vi "ELL9 Device Engine.vi"() -> ()   [LabVIEW 2020]
uses:
  FW Type Defs/FW Actions.ctl
  FW Type Defs/FW Notifier Type.ctl
  <vilib>/Instr/_visa.llb/VISA Configure Serial Port (Instr).vi
panel:
  out "FW ID":string
  in  "COM Port":string[](array[string])
  in  "Notifier Name":string="Not a Name"
  out "Current Position":u8
  in  "Quit":bool
  in  "Get Position":bool
  in  "FW Position":u8=1 min=1 max=8
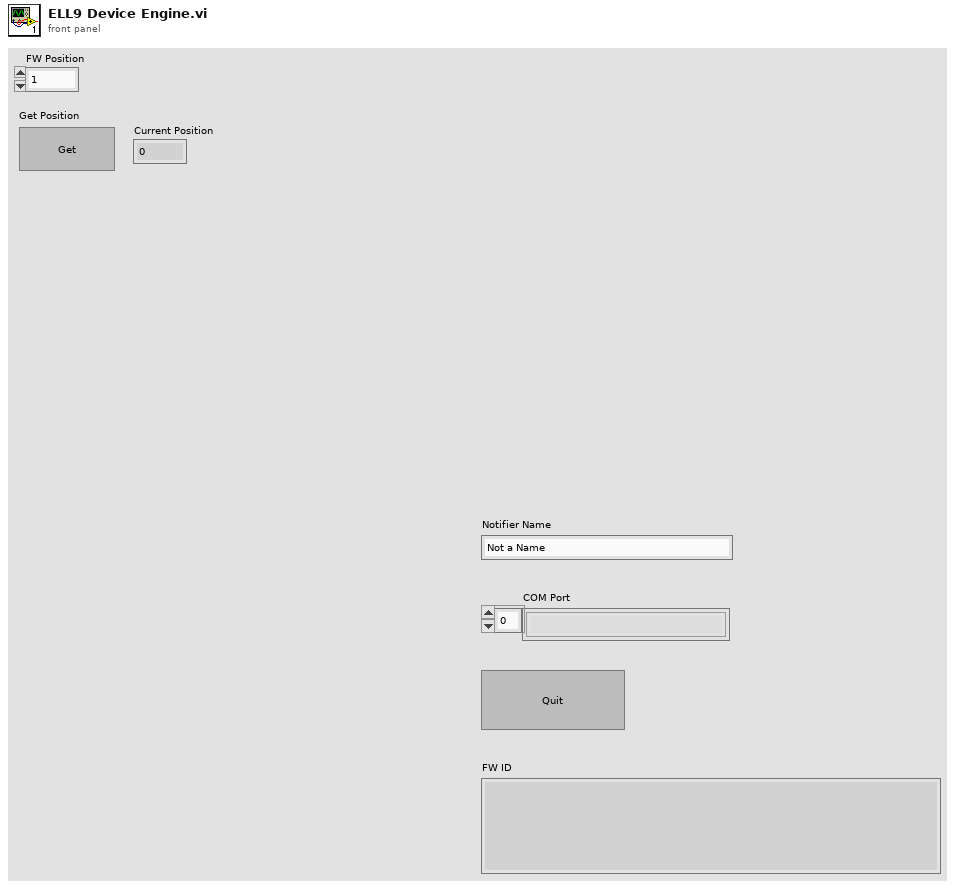
[diagram p1: front panel]
types:
  T1 = typedef "FW Notifier Type.ctl" = cluster{"Actions":T2, "Set Position":u8, "Actual Position":u8, "Speed":dbl, "Num Positions":u8, "Received":bool}
  T2 = typedef "FW Actions.ctl" = enum16{"Set Position", "Get Position", "Get Num Positions", "Set Speed", "Confirm Pos", "Quit"}
  T3 = enum32{"Invalid", "Standard", "Closed", "Hidden", "Minimized", "Maximized"}
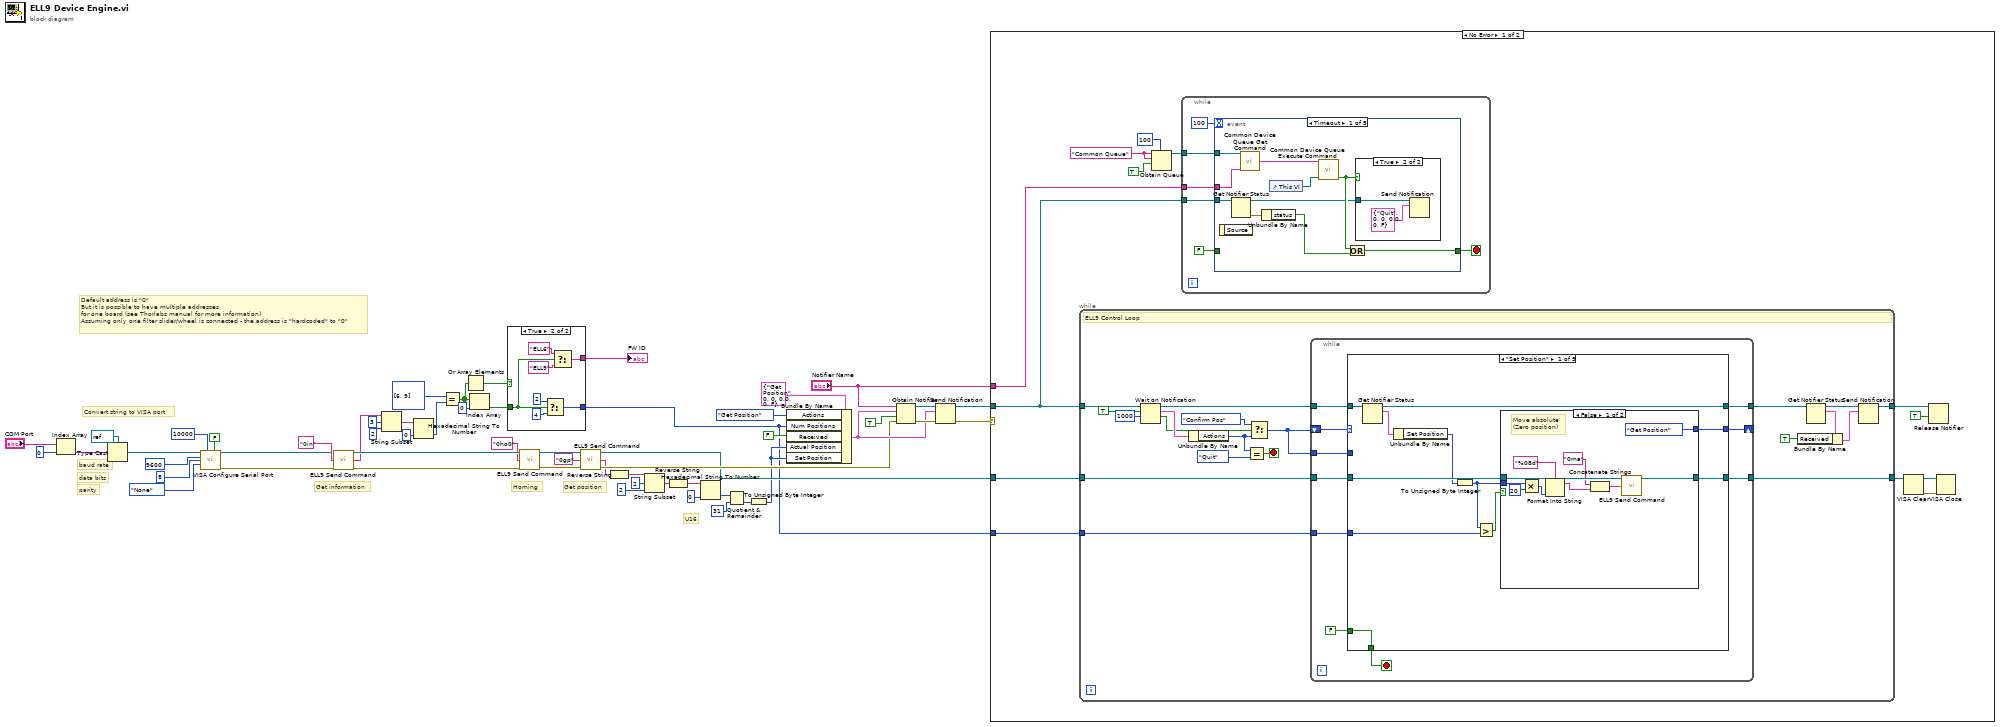
[diagram p0: block diagram]
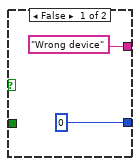
[diagram p2: hidden frame]
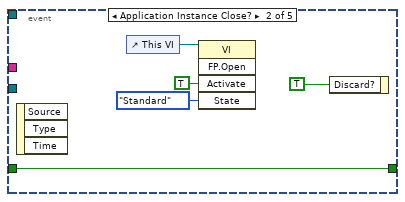
[diagram p4: hidden frame]
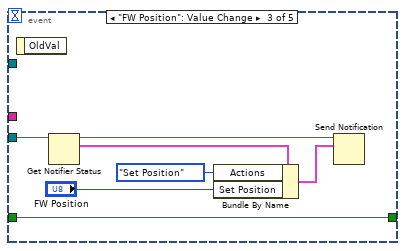
[diagram p5: hidden frame]
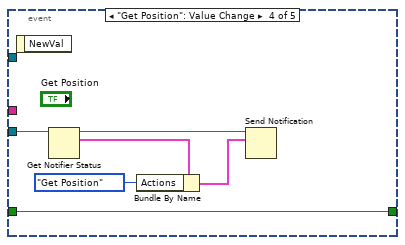
[diagram p6: hidden frame]
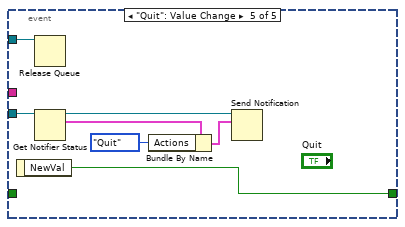
[diagram p7: hidden frame]
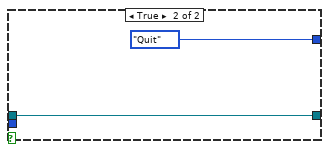
[diagram p8: hidden frame]
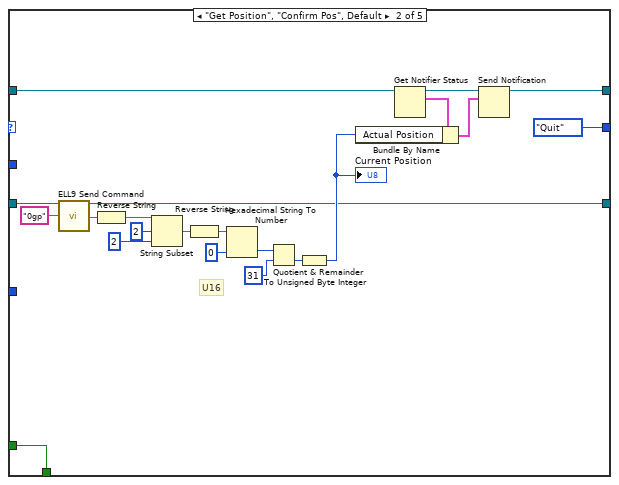
[diagram p9: hidden frame]
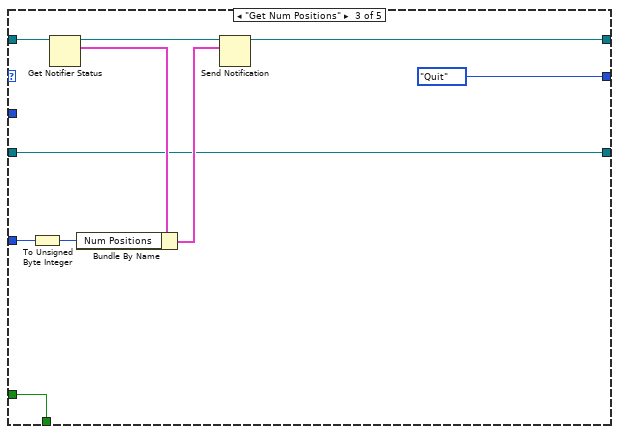
[diagram p10: hidden frame]
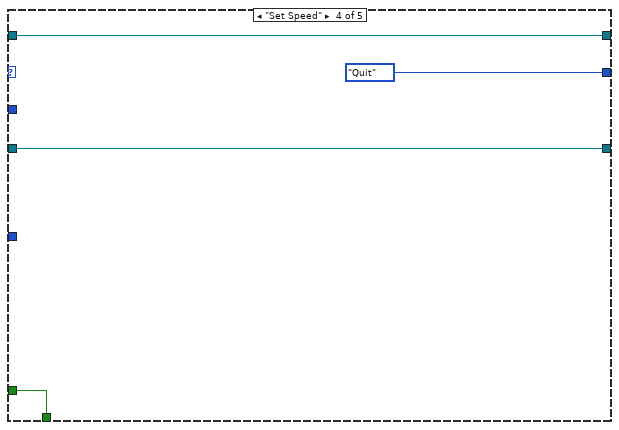
[diagram p11: hidden frame]
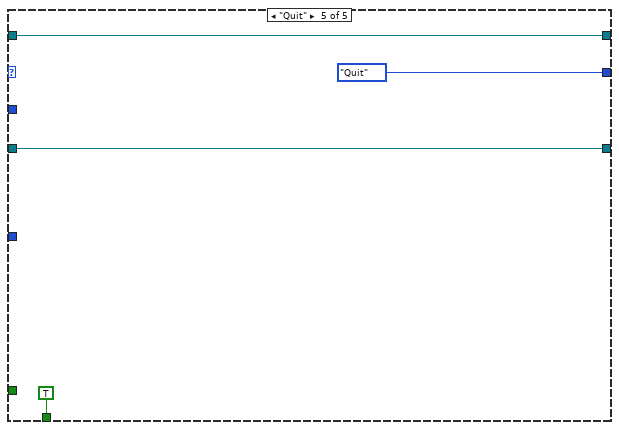
[diagram p12: hidden frame]
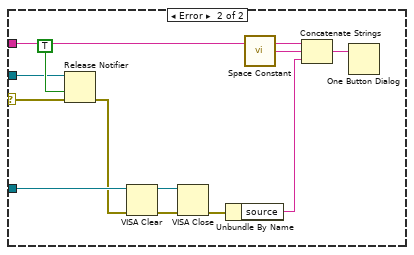
[diagram p13: hidden frame]
diagram:
  # "U16"
  # "Get position"
  # "Default address is \"0\"\nBut it is possible to have multiple addresses \nfor one board (see Thorlabs manual for more information)\nAssuming only one filter slider/wheel is connected - the address is \"hardcoded\" to \"0\""
  # "Get information"
  # "Homing"
  # "Convert string to VISA port"
  # "parity"
  # "data bits"
  # "baud rate"
  n1 = Index Array(array="COM Port", index=0) -> (element=w38:string)
  n2 = Type Cast(type=refnum<visa-resource-name> refnum ("VISA resource name"), x=w38) -> (*(type *) &x=w36:refnum<visa-resource-name>)
  n3 = call-poly "VISA Configure Serial Port"("VISA resource name"=w36, "timeout (10sec)"=u32 10000, "Enable Termination\nChar (T)"=FALSE ("Enable Termination\nChar (T)"), "baud rate (9600)"=u32 9600 ("nbaud"), "data bits (8)"=u16 8, "parity (0:none)"=enum16{"None", "Odd", "Even", "Mark", "Space"}."None") -> ("VISA resource name out"=w27:refnum<visa-resource-name>, "error out"=w1:errorcluster)  [unwired: 4 in, 4 out]
  n4 = call "ELL9 Send Command.vi"("VISA Ref"=w27, "Command"="0in" ("write buffer"), "Error In"=w1) -> ("VISA Ref Dup"=w33:refnum<visa-resource-name>, "Reply"=w5:string, "Error Out"=w34:errorcluster)  [unwired: 9 in, 1 out]
  n5 = String Subset(string=w5, offset (0)=3, length (rest)=2 ("length (rest)")) -> (substring=w11:string)
  n6 = Hexadecimal String To Number(string=w11, default (0uL)=u16 0 ("default (0 U32)")) -> (number=w4:u16)  [unwired: 1 in, 1 out]
  n7 = Equal?(x=u16[] [6, 9] ("default (0 U32)"), y=w4) -> (x = y?=w9:bool[])
  n8 = Or Array Elements(Boolean array=w9) -> (logical OR=w10:bool)
  n9 = Index Array(array=w9, index=0) -> (element=w7:bool)
  n10 = case shown="True" w10 {
    tunnel: w7 -> [_ w61]
    tunnel: ["Wrong device" ("write buffer") w62] -> w6
    tunnel: [u8 0 ("default (0 U32)") w58] -> w2
    frame False {
    }
    frame True {
      n11 = Select(t=u8 2 ("default (0 U32)"), s=w61, f=u8 4 ("default (0 U32)")) -> (s? t:f=w58:u8)
      n12 = Select(t="ELL6" ("write buffer"), s=w61, f="ELL9" ("write buffer")) -> (s? t:f=w62:string)
    }
  }
  "FW ID" <- w6
  n13 = call "ELL9 Send Command.vi"("VISA Ref"=w33, "Command"="0ho0" ("write buffer"), "Error In"=w34) -> ("VISA Ref Dup"=w30:refnum<visa-resource-name>, "Error Out"=w31:errorcluster)  [unwired: 9 in, 2 out]
  n14 = call "ELL9 Send Command.vi"("VISA Ref"=w30, "Command"="0gp" ("write buffer"), "Error In"=w31) -> ("VISA Ref Dup"=w21:refnum<visa-resource-name>, "Reply"=w24:string, "Error Out"=w28:errorcluster)  [unwired: 9 in, 1 out]
  n15 = Reverse String(1:w24) -> (0:w23:string)
  n16 = String Subset(string=w23, offset (0)=2, length (rest)=2 ("length (rest)")) -> (substring=w22:string)
  n17 = Reverse String(1:w22) -> (0:w18:string)
  n18 = Hexadecimal String To Number(string=w18, default (0uL)=u16 0 ("default (0 U32)")) -> (number=w20:u16)  [unwired: 1 in, 1 out]
  n19 = Quotient & Remainder(x=w20, y=u16 31) -> (floor(x/y)=w16:u16)  [unwired: 1 out]
  n20 = To Unsigned Byte Integer(number=w16) -> (unsigned 8bit integer=w15:u8)
  n21 = Bundle By Name(cluster=T1 {"Actions"=enum."Get Position", "Set Position"=0, "Actual Position"=0, "Speed"=0.0, "Num Positions"=0, "Received"=FALSE} ("Note Type"), "Actions"=FW_Actions."Get Position", "Num Positions"=w2, "Received"=FALSE ("Received?"), "Actual Position"=w15, "Set Position"=w15) -> (w49:T1)
  n22 = Obtain Notifier(name (unnamed)="Notifier Name", notification data type=w49, create if not found? (T)=TRUE, error in (no error)=w28) -> (notifier out=w54:refnum<notifier>, error out=w53:errorcluster)  [unwired: 1 out]
  n23 = Send Notification(notification=w49, notifier=w54, error in (no error)=w53) -> (notifier out=w47:refnum<notifier>, error out=w48:errorcluster)
  n24 = case shown="No Error" w48 {
    selector: w48 -> [_ w222]
    tunnel: w47 -> [w75 w223]
    tunnel: "Notifier Name" -> [w74 w221]
    tunnel: w21 -> [w69 w214]
    tunnel: w2 -> [w68 _]
    frame No Error {
      w73 = "Common Queue" ("Unique Notifier Name")
      n25 = while {
        tunnel: w75 -> [w134]
        tunnel: [w135] -> w76
        tunnel: w69 -> [w130]
        tunnel: [w129] -> w65
        tunnel: w68 -> [w128]
        stop <- w140 stop-if-true
        # "ELL9 Control Loop"
        n26 = Wait on Notification(notifier=w134, ignore previous (F)=TRUE, timeout in ms (-1)=1000) -> (notifier out=w132:refnum<notifier>, notification=w127:T1, timed out?=w123:bool)  [unwired: 1 in, 1 out]
        n27 = Unbundle By Name(w127) -> ("Actions"=w124:T2)
        n28 = Equal?(x=w124, y=FW_Actions."Quit") -> (x = y?=w140:bool)
        n29 = Select(t=FW_Actions."Confirm Pos", s=w123, f=w124) -> (s? t:f=w122:T2)
        n30 = while {
          tunnel: w132 -> [w149]
          tunnel: [w148] -> w131
          tunnel: w130 -> [w145]
          tunnel: [w144] -> w129
          tunnel: w128 -> [w143]
          shift-right: [w142] -> _
          shift-left: w122 -> [w150]
          tunnel: w122 -> [w141]
          stop <- w146 stop-if-true
          n31 = case shown="\"Set Position\"" w150 {
            tunnel: w149 -> [w157 w193 w203 w208 w212]
            tunnel: [w156 w191 w201 w208 w212] -> w148
            tunnel: [w161 w194 w204 w206 TRUE] -> w146
            tunnel: FALSE -> [w161 w194 w204 w206 _]
            tunnel: w145 -> [w159 w187 w195 w205 w210]
            tunnel: [w155 w174 w195 w205 w210] -> w144
            tunnel: w143 -> [w152 _ w198 _ _]
            tunnel: [w160 FW_Actions."Quit" ("f") FW_Actions."Quit" ("f") FW_Actions."Quit" ("f") FW_Actions."Quit" ("f")] -> w142
            tunnel: w141 -> [_ _ _ _ _]
            frame "Set Position" {
              n32 = Get Notifier Status(notifier=w157) -> (notifier out=w156:refnum<notifier>, current notification=w158:T1)  [unwired: 1 in, 3 out]
              n33 = Unbundle By Name(w158) -> ("Set Position"=w154:u8)
              n34 = To Unsigned Byte Integer(number=w154) -> (unsigned 8bit integer=w153:u8)
              n35 = Greater?(x=w153, y=w152) -> (0:w151:bool)
              n36 = case shown="False" w151 {
                tunnel: [FW_Actions."Get Position" ("f") FW_Actions."Quit" ("f")] -> w160
                tunnel: w159 -> [w170 w173]
                tunnel: [w169 w173] -> w155
                tunnel: w153 -> [w168 _]
                frame False {
                  # "Move absolute\n(Zero position)"
                  n37 = Multiply(x=w168, y=u8 20) -> (x*y=w165:u8)
                  n38 = Format Into String(format string="%08d", w165) -> (resulting string=w164:string)  [unwired: 2 in, 1 out]
                  n39 = Concatenate Strings("0ma", w164) -> (w162:string)
                  n40 = call "ELL9 Send Command.vi"("VISA Ref"=w170, "Command"=w162) -> ("VISA Ref Dup"=w169:refnum<visa-resource-name>)  [unwired: 10 in, 3 out]
                }
                frame True {
                }
              }
            }
            frame "Get Position", "Confirm Pos", Default {
              # "U16"
              n41 = call "ELL9 Send Command.vi"("VISA Ref"=w187, "Command"="0gp" ("write buffer")) -> ("VISA Ref Dup"=w174:refnum<visa-resource-name>, "Reply"=w176:string)  [unwired: 10 in, 2 out]
              n42 = Reverse String(1:w176) -> (0:w183:string)
              n43 = String Subset(string=w183, offset (0)=2, length (rest)=2 ("length (rest)")) -> (substring=w182:string)
              n44 = Reverse String(1:w182) -> (0:w179:string)
              n45 = Hexadecimal String To Number(string=w179, default (0uL)=u16 0 ("default (0 U32)")) -> (number=w181:u16)  [unwired: 1 in, 1 out]
              n46 = Quotient & Remainder(x=w181, y=u16 31) -> (floor(x/y)=w177:u16)  [unwired: 1 out]
              n47 = To Unsigned Byte Integer(number=w177) -> (unsigned 8bit integer=w175:u8)
              "Current Position" <- w175
              n48 = Get Notifier Status(notifier=w193) -> (notifier out=w192:refnum<notifier>, current notification=w190:T1)  [unwired: 1 in, 3 out]
              n49 = Bundle By Name(cluster=w190, "Actual Position"=w175) -> (w189:T1)
              n50 = Send Notification(notification=w189, notifier=w192) -> (notifier out=w191:refnum<notifier>)  [unwired: 1 in, 1 out]
            }
            frame "Get Num Positions" {
              n51 = To Unsigned Byte Integer(number=w198) -> (unsigned 8bit integer=w197:u8)
              n52 = Get Notifier Status(notifier=w203) -> (notifier out=w202:refnum<notifier>, current notification=w199:T1)  [unwired: 1 in, 3 out]
              n53 = Bundle By Name(cluster=w199, "Num Positions"=w197) -> (w196:T1)
              n54 = Send Notification(notification=w196, notifier=w202) -> (notifier out=w201:refnum<notifier>)  [unwired: 1 in, 1 out]
            }
            frame "Set Speed" {
            }
            frame "Quit" {
            }
          }
        }
        n55 = Get Notifier Status(notifier=w131) -> (notifier out=w136:refnum<notifier>, current notification=w138:T1)  [unwired: 1 in, 3 out]
        n56 = Bundle By Name(cluster=w138, "Received"=TRUE ("Received?")) -> (w139:T1)
        n57 = Send Notification(notification=w139, notifier=w136) -> (notifier out=w135:refnum<notifier>)  [unwired: 1 in, 1 out]
      }
      n58 = Obtain Queue(max queue size (-1, unlimited)=100, name (unnamed)=w73, element data type=w73, create if not found? (T)=TRUE) -> (queue out=w70:refnum<queue>)  [unwired: 1 in, 2 out]
      n59 = while {
        tunnel: w70 -> [w83]
        tunnel: w75 -> [w80]
        tunnel: w74 -> [w78]
        stop <- w79 stop-if-true
        n60 = event shown="[0] Timeout" {
          selector: _ -> [_ _ _ _ _]
          dyn-events: _ -> [_ _ _ _ _]
          timeout: 100 -> [_ _ _ _ _]
          tunnel: w83 -> [w91 _ _ _ w116]
          tunnel: FALSE -> [_ w100 w107 w113 _]
          tunnel: w80 -> [w93 _ w106 w112 w117]
          tunnel: [w86 w100 w107 w113 w120] -> w79
          tunnel: w78 -> [w90 _ _ _ _]
          event Timeout {
            n61 = event-data() -> ()  [unwired: 1 in, 1 out]
            n62 = Get Notifier Status(notifier=w93) -> (notifier out=w84:refnum<notifier>, error out=w92:errorcluster)  [unwired: 1 in, 3 out]
            n63 = call "Common Device Queue Get Command.vi"("Common Queue"=w91, "Notifier Name"=w90) -> ("Command"=w89:string)  [unwired: 12 in, 1 out]
            n64 = Unbundle By Name(w92) -> ("status"=w87:bool)
            n65 = control-ref of="This VI"() -> (w88:refnum<vi>)
            n66 = call "Common Device Queue Execute Command.vi"("Common Command"=w89, "VI Refnum"=w88) -> ("Quit?"=w85:bool)  [unwired: 12 in, 1 out]
            n67 = Or(x=w85, y=w87) -> (x .or. y?=w86:bool)
            n68 = case shown="True" w85 {
              tunnel: w84 -> [_ w95]
              frame False {
              }
              frame True {
                n69 = Send Notification(notification=T1 {"Actions"=enum."Quit", "Set Position"=0, "Actual Position"=0, "Speed"=0.0, "Num Positions"=0, "Received"=FALSE} ("Note Type"), notifier=w95) -> ()  [unwired: 1 in, 2 out]
              }
            }
          }
          event Application Instance Close? {
            n70 = event-data() -> ()  [unwired: 1 in, 3 out]
            n71 = control-ref of="This VI"() -> (w97:refnum<vi>)
            n72 = invoke class="VI" method="FP.Open"(reference=w97, "Activate"=TRUE ("Activate?"), "State"=T3."Standard") -> ()  [unwired: 2 in, 5 out]
            n73 = event-data("Discard?"=TRUE) -> ()  [unwired: 1 in, 1 out]
          }
          event "FW Position": Value Change {
            n74 = event-data() -> ()  [unwired: 1 in, 1 out]
            n75 = Get Notifier Status(notifier=w106) -> (notifier out=w105:refnum<notifier>, current notification=w104:T1)  [unwired: 1 in, 3 out]
            n76 = Bundle By Name(cluster=w104, "Actions"=FW_Actions."Set Position", "Set Position"="FW Position") -> (w103:T1)
            n77 = Send Notification(notification=w103, notifier=w105) -> ()  [unwired: 1 in, 2 out]
          }
          event "Get Position": Value Change {
            n78 = event-data() -> ()  [unwired: 1 in, 1 out]
            n79 = Get Notifier Status(notifier=w112) -> (notifier out=w111:refnum<notifier>, current notification=w110:T1)  [unwired: 1 in, 3 out]
            n80 = Bundle By Name(cluster=w110, "Actions"=FW_Actions."Get Position") -> (w109:T1)
            n81 = Send Notification(notification=w109, notifier=w111) -> ()  [unwired: 1 in, 2 out]
          }
          event "Quit": Value Change {
            n82 = event-data() -> ("NewVal"=w120:bool)  [unwired: 1 in]
            n83 = Release Queue(queue=w116) -> ()  [unwired: 2 in, 3 out]
            n84 = Get Notifier Status(notifier=w117) -> (notifier out=w119:refnum<notifier>, current notification=w115:T1)  [unwired: 1 in, 3 out]
            n85 = Bundle By Name(cluster=w115, "Actions"=FW_Actions."Quit") -> (w118:T1)
            n86 = Send Notification(notification=w118, notifier=w119) -> ()  [unwired: 1 in, 2 out]
          }
        }
      }
      n87 = VISA Clear(VISA resource name=w65) -> (VISA resource name out=w66:refnum<visa-resource-name>, error out=w67:errorcluster)  [unwired: 1 in]
      n88 = Release Notifier(notifier=w76, force destroy? (F)=TRUE) -> ()  [unwired: 1 in, 3 out]
      n89 = VISA Close(VISA resource name=w66, error in (no error)=w67) -> ()  [unwired: 1 out]
    }
    frame Error {
      n90 = Release Notifier(notifier=w223, force destroy? (F)=TRUE, error in (no error)=w222) -> (error out=w213:errorcluster)  [unwired: 2 out]
      n91 = VISA Clear(VISA resource name=w214, error in (no error)=w213) -> (VISA resource name out=w216:refnum<visa-resource-name>, error out=w217:errorcluster)
      n92 = VISA Close(VISA resource name=w216, error in (no error)=w217) -> (error out=w215:errorcluster)
      n93 = Unbundle By Name(w215) -> ("source"=w218:string)
      n94 = call <vilib>:"Space Constant.vi"() -> ("String"=w219:string)
      n95 = Concatenate Strings(w221, w219, w218) -> (w220:string)
      n96 = One Button Dialog(message=w220) -> ()  [unwired: 1 in, 1 out]
    }
  }
